vi "Analog_Delay.vi"(8 "Time":dbl=-1.0, 9 "Delay Time":dbl=1.0, 11 "Input":dbl) -> (1 "IsPresent":bool, 3 "Output":dbl)   [LabVIEW 2019, in "Trajectory_Library.lvlib"]
doc: "This VI implements an analog \"time delay\". The output is the input delayed by \"Delay\" seconds. If the \"Delay\" time does not exactly match the sample period,, the value is calculated by interpolating the nearest buffer samples.\n\nInputs:\n - Input -- Double input value\n - Delay Time -- Time (seconds) to delay the otuput value. If time delay is increaed, then the buffer is re-created. FALSE will be returned until the buffer has sufficient data to return a delayed value.\n - Time -- Continously counting system time, Seconds. If not wired the FPGA time will be used.\n\nOutputs:\n - Output -- Double output value with delay applied\n - IsPresent -- Set to TRUE if the buffer has enough data to return a delayed value."
uses:
  Trajectory_Library.lvlib
  TimeInterpDouble_CleanUp.vi
  MathUtil_Interpolate.vi
  MathUtil_Clamp.vi
  <vilib>/gmath/interp.llb/Search Ordered Table.vi
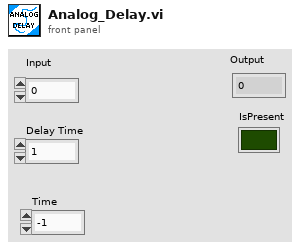
[diagram p1: front panel]
types:
  T1 = typedef "Trajectory_Library.lvlib/TIME_INTERPOLATABLE_DOUBLE.ctl" = cluster{"TimeStamps":dbl[], "DoubleValue":dbl[], "Min_TimeStamp":dbl, "Max_TimeStamp":dbl, "ItemCount":i32, "MaxBufferTime":dbl}
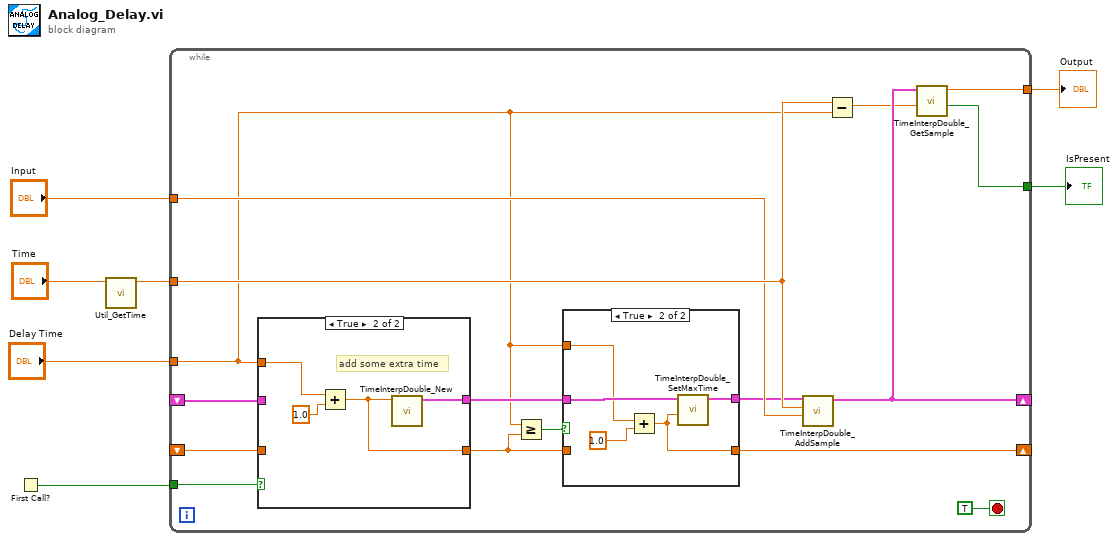
[diagram p0: block diagram]
diagram:
  n1 = First Call?() -> (First Call?: T/F=w6:bool)
  n2 = call "Util_GetTime.vi"("Pass_Through_Time"="Time") -> ("FPGA_Time_Seconds"=w4:dbl)  [unwired: 9 in, 1 out]
  n3 = while {
    tunnel: "Delay Time" -> [w8]
    tunnel: w6 -> [w14]
    shift-right: [w22] -> _
    shift-left: _ -> [w17]
    tunnel: w4 -> [w21]
    tunnel: "Input" -> [w15]
    tunnel: [w19] -> w2
    tunnel: [w18] -> w1
    shift-right: [w11] -> _
    shift-left: _ -> [w16]
    stop <- TRUE stop-if-true
    n4 = case shown="True" w14 {
      tunnel: w8 -> [_ w34]
      tunnel: [w32 w35] -> w13
      tunnel: w17 -> [w32 _]
      tunnel: [w31 w33] -> w9
      tunnel: w16 -> [w31 _]
      frame False {
      }
      frame True {
        # "add some extra time"
        n5 = Add(x=w34, y=1.0) -> (x+y=w33:dbl)
        n6 = call "TimeInterpDouble_New.vi"("MaxTime"=w33) -> ("TimeInterpDouble"=w35:T1)  [unwired: 10 in]
      }
    }
    n7 = Greater Or Equal?(x=w8, y=w9) -> (x >= y?=w10:bool)
    n8 = case shown="True" w10 {
      tunnel: w13 -> [w25 w30]
      tunnel: w8 -> [_ w28]
      tunnel: [w25 w27] -> w12
      tunnel: [w24 w26] -> w11
      tunnel: w9 -> [w24 _]
      frame False {
      }
      frame True {
        n9 = Add(x=w28, y=1.0) -> (x+y=w26:dbl)
        n10 = call "TimeInterpDouble_SetMaxTime.vi"("Max Time"=w26, "in TimeInterpDouble"=w30) -> ("out TimeInterpDouble"=w27:T1)  [unwired: 9 in]
      }
    }
    n11 = call "TimeInterpDouble_AddSample.vi"("Value"=w15, "TimeStamp"=w21, "in TimeInterpDouble"=w12) -> ("out TimeInterpDouble"=w22:T1)  [unwired: 7 in, 1 out]
    n12 = Subtract(x=w21, y=w8) -> (x-y=w20:dbl)
    n13 = call "TimeInterpDouble_GetSample.vi"("TimeStamp"=w20, "TimeInterpDouble"=w22) -> ("IsPresent"=w18:bool, "OutputDouble"=w19:dbl)  [unwired: 8 in]
  }
  "Output" <- w2
  "IsPresent" <- w1
